vi "checkCmdOrEvent.vi"(8 "error in (no error)":errorcluster, 10 "tcpPacket":string, 11 "tcpServerCmd in":refnum<class "TcpServerCmd.lvclass">) -> (0 "error out":errorcluster, 2 "typeOfPacket":string, 3 "tcpServerCmd out":refnum<class "TcpServerCmd.lvclass">)   [LabVIEW 2018, in "TcpServerCmd.lvclass"]
doc: "Check if the incoming packet is a command or an event. In other case, it will define the type of packet as \"unknown\"."
uses:
  TcpServerCmd.lvclass
  <vilib>/regexp/Match Regular Expression.xnode
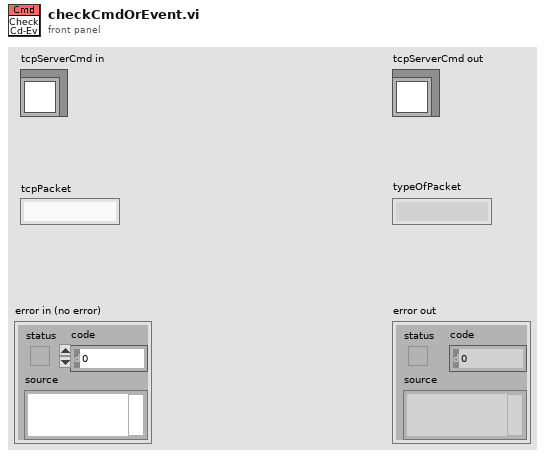
[diagram p1: front panel]
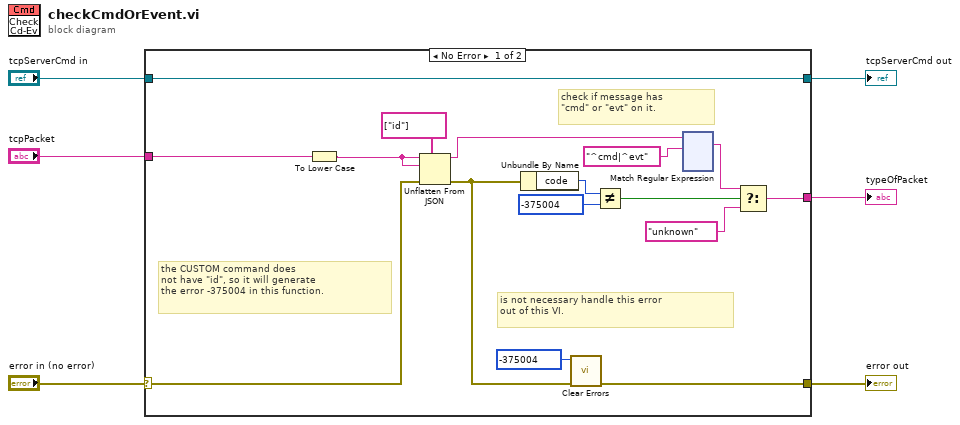
[diagram p0: block diagram]
diagram:
  n1 = case shown="No Error" "error in (no error)" {
    selector: "error in (no error)" -> [w16 w138]
    tunnel: [w13 w138] -> w5
    tunnel: [w8 w137] -> w4
    tunnel: [w12 _] -> w3
    tunnel: "tcpServerCmd in" -> [w8 w137]
    tunnel: "tcpPacket" -> [w7 _]
    frame No Error {
      # "check if message has\n\"cmd\" or \"evt\" on it."
      # "the CUSTOM command does\nnot have \"id\", so it will generate\nthe error -375004 in this function."
      # "is not necessary handle this error\nout of this VI."
      n2 = To Lower Case(string=w7) -> (all lower case string=w17:string)
      n3 = Unflatten From JSON(path=string[] ["id"], JSON string=w17, type and defaults=w17, error in (no error)=w16) -> (value=w11:string, error out=w14:errorcluster)  [unwired: 3 in]
      n4 = Unbundle By Name(w14) -> ("code"=w21:i32)
      n5 = call <vilib>:"Clear Errors.vi"("error in (no error)"=w14, "specific error code to clear (0: all)"=-375004) -> ("error out"=w13:errorcluster)  [unwired: 4 in, 1 out]
      n6 = Not Equal?(x=w21, y=-375004) -> (x != y?=w19:bool)
      n7 = xnode "Match Regular Expression"("input string"=w11, "regular expression"="^cmd|^evt") -> ("whole match"=w9:string)  [unwired: 4 in, 4 out]
      n8 = Select(t=w9, s=w19, f="unknown" ("t")) -> (s? t:f=w12:string)
    }
    frame Error {
    }
  }
  "error out" <- w5
  "tcpServerCmd out" <- w4
  "typeOfPacket" <- w3
